vi "Higher_Level_subVIs_example_circ_buffer.vi"() -> ()   [LabVIEW 2021]
panel:
  in  "stop":bool
  out "Intensity Graph":dbl[][](graph)
  out "image buff 2":u16[](array[numeric])
  out "Data (no BG subtracted)":u16[][](array[numeric])
  out "Temp (C)":dbl
  out "image buff":u16[](array[numeric])
  out "Array":string[](array[string])
  in  "Exposure (ms)":dbl=100.0
  out "Camera Error":errorcluster
  in  "Exposure Time (s)":dbl(slide) min=1.0 max=62.0 step=1.0 scale=0.005..10.0
  out "Camera Handle":i16
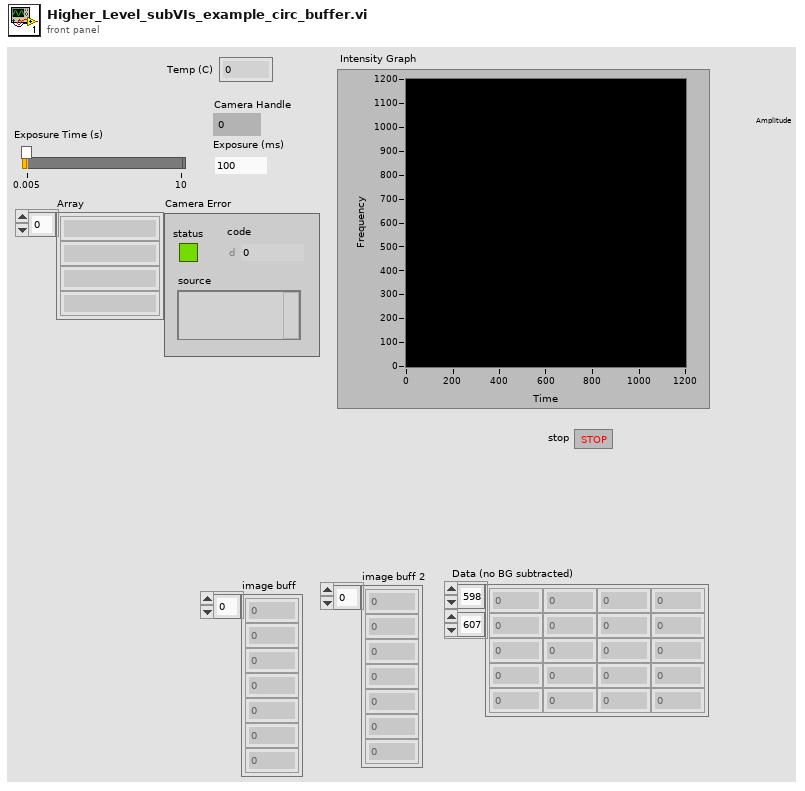
[diagram p1: front panel]
types:
  T1 = enum16{"CCS_NO_CHANGE", "CCS_HALT", "CCS_HALT_CLOSE_SHTR", "CCS_CLEAR", "CCS_CLEAR_CLOSE_SHTR", "CCS_OPEN_SHTR", "CCS_CLEAR_OPEN_SHTR"}
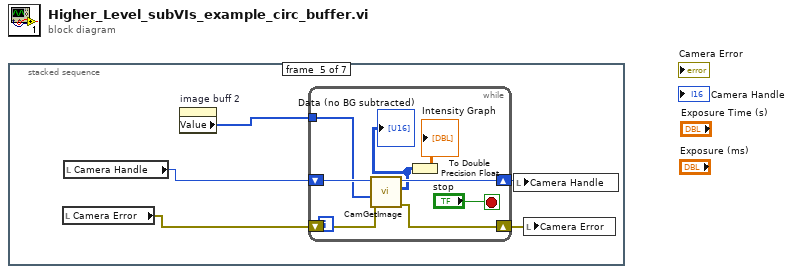
[diagram p0: block diagram]
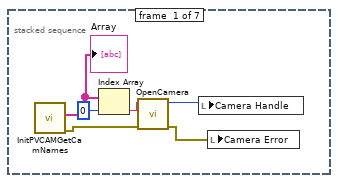
[diagram p2: hidden frame]
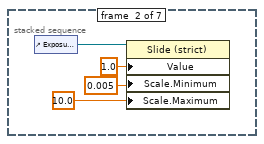
[diagram p3: hidden frame]
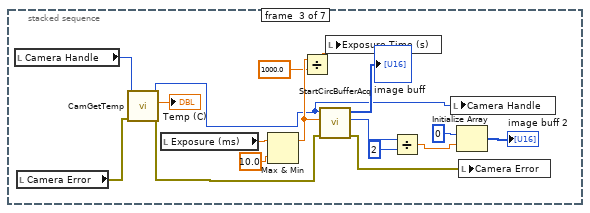
[diagram p4: hidden frame]
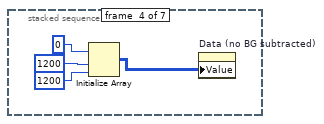
[diagram p5: hidden frame]
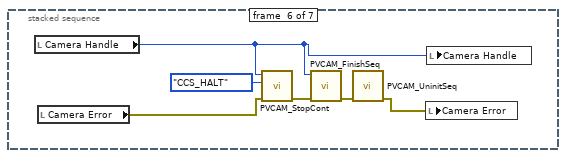
[diagram p6: hidden frame]
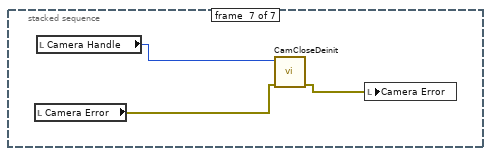
[diagram p7: hidden frame]
diagram:
  n1 = stacked-sequence {
    frame #0 {
      n2 = call "InitPVCAMGetCamNames.vi"() -> ("error out"=w3:errorcluster, "Array"=w6:string[])  [unwired: 8 in, 1 out]
      "Array" <- w6
      n3 = Index Array(array=w6, index=0) -> (element=w4:string)
      n4 = call "OpenCamera.vi"("error in (no error)"=w3, "cameraName"=w4) -> ("error out"=w1:errorcluster, "hCam out"=w2:i16)  [unwired: 6 in, 1 out]
      n5 = local write "Camera Handle"(w2) -> ()
      n6 = local write "Camera Error"(w1) -> ()
    }
    frame #1 {
      n7 = control-ref of="Exposure Time (s)"() -> (w10:refnum<vi>)
      n8 = property on="Property Node" class="Slide (strict)"(reference=w10, "Value"=1.0, "Scale.Minimum"=0.005 ("Scale.Range:Minimum"), "Scale.Maximum"=10.0 ("Scale.Range:Maximum")) -> ()  [unwired: 1 in, 2 out]
    }
    frame #2 {
      n9 = local read "Camera Handle"() -> (w14:i16)
      n10 = local read "Camera Error"() -> (w11:errorcluster)
      n11 = call "CamGetTemp.vi"("error in (no error)"=w11, "hCam"=w14) -> ("error in (no error) 2"=w12:errorcluster, "temperature"=→"Temp (C)":dbl, "hCam out"=w13:i16)  [unwired: 7 in]
      n12 = local read "Exposure (ms)"() -> (w24:dbl)
      n13 = Max & Min(x=w24, y=10.0) -> (max(x,y)=w18:dbl)  [unwired: 1 out]
      n14 = Divide(x=w18, y=1000.0) -> (x/y=w16:dbl)
      n15 = call "StartCircBufferAcq.vi"("error in (no error)"=w12, "exp_time"=w18, "hCam"=w13) -> ("error out"=w25:errorcluster, "stream_size"=w21:u32, "image buff"=→"image buff":u16[])  [unwired: 6 in]
      n16 = local write "Exposure Time (s)"(w16) -> ()
      n17 = Divide(x=w21, y=u32 2) -> (x/y=w19:dbl)
      n18 = local write "Camera Handle"(w13) -> ()
      n19 = Initialize Array(i16 0 ("element"), w19) -> (→"image buff 2":i16[])
      n20 = local write "Camera Error"(w25) -> ()
    }
    frame #3 {
      n21 = Initialize Array(i16 0 ("dimension size"), 1200 ("dimension size"), 1200 ("dimension size")) -> (w28:i16[][])
      n22 = property on="Data (no BG subtracted)" class="Arr (strict)"("Value"=w28) -> ()  [unwired: 2 in, 2 out]
    }
    frame #4 {
      n23 = local read "Camera Error"() -> (w32:errorcluster)
      n24 = local read "Camera Handle"() -> (w33:i16)
      n25 = property on="image buff 2" class="Arr (strict)"() -> ("Value"=w34:u16[])  [unwired: 2 in, 2 out]
      n26 = while {
        tunnel: w34 -> [w40]
        shift-right: [w42] -> w36
        shift-left: w33 -> [w44]
        shift-right: [w41] -> w35
        shift-left: w32 -> [w43]
        stop <- "stop" stop-if-true
        n27 = call "CamGetImage.vi"("error in (no error)"=w43, "buffer for frame"=w40, "hCam"=w44) -> ("error out"=w41:errorcluster, "output array"=w39:u16[][], "hCam out"=w42:i16)  [unwired: 6 in]
        "Data (no BG subtracted)" <- w39
        n28 = To Double Precision Float(number=w39) -> (double precision float=→"Intensity Graph":dbl[][])
      }
      n29 = local write "Camera Handle"(w36) -> ()
      n30 = local write "Camera Error"(w35) -> ()
    }
    frame #5 {
      n31 = local read "Camera Handle"() -> (w45:i16)
      n32 = local read "Camera Error"() -> (w47:errorcluster)
      n33 = call "PVCAM_StopCont.vi"("error in (no error)"=w47, "cam_state"=T1."CCS_HALT", "hCam"=w45) -> ("error out"=w50:errorcluster)  [unwired: 7 in, 1 out]
      n34 = call "PVCAM_FinishSeq.vi"("error in (no error)"=w50, "hCam"=w45) -> ("error out"=w49:errorcluster)  [unwired: 8 in, 1 out]
      n35 = call "PVCAM_UninitSeq.vi"("error in (no error)"=w49) -> ("error out"=w46:errorcluster)  [unwired: 9 in, 1 out]
      n36 = local write "Camera Error"(w46) -> ()
      n37 = local write "Camera Handle"(w45) -> ()
    }
    frame #6 {
      n38 = local read "Camera Error"() -> (w52:errorcluster)
      n39 = local read "Camera Handle"() -> (w51:i16)
      n40 = call "CamCloseDeinit.vi"("error in (no error)"=w52, "hCam"=w51) -> ("error out"=w53:errorcluster)  [unwired: 9 in]
      n41 = local write "Camera Error"(w53) -> ()
    }
  }
